vi "getMessage.vi"(8 "error in (no error)":errorcluster, 11 "SerialCommunicator in":refnum<class "SerialCommunicator.lvclass">) -> (0 "error out":errorcluster, 2 "String":string, 3 "SerialCommunicator out":refnum<class "SerialCommunicator.lvclass">)   [LabVIEW 2016, in "SerialCommunicator.lvclass"]
uses:
  SerialCommunicator.lvclass
  Communicator/Communicator.lvclass
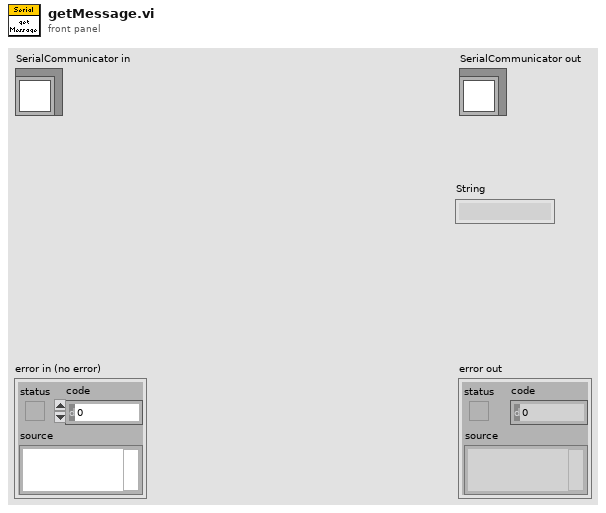
[diagram p1: front panel]
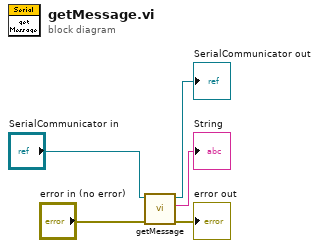
[diagram p0: block diagram]
diagram:
  n1 = call-parent "getMessage.vi"("error in (no error)"="error in (no error)", "Communicator in"="SerialCommunicator in") -> ("error out"=→"error out":errorcluster, "String"=→"String":string, "Communicator out"=→"SerialCommunicator out":refnum<class "SerialCommunicator.lvclass">)  [unwired: 7 in]
